vi "To Array U16 1D.vi"(8 "error in":errorcluster, 11 "Generic Image in":refnum<class "Generic Image.lvclass">) -> (0 "error out":errorcluster, 1 "Timestamp":timestamp, 2 "U16":u16[](array[numeric]))   [LabVIEW 2025, in "Generic Image.lvclass"]
uses:
  Generic Image.lvclass
  Generic Image.lvclass/Generic Image.ctl
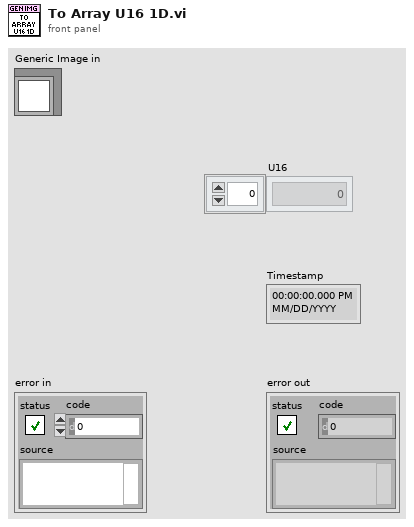
[diagram p1: front panel]
types:
  T1 = typedef "Generic Image.lvclass/Pixel Format.ctl" = enum16{"Grayscale (U8)", "Grayscale (I16)", "Grayscale (SGL)", "Complex (CSG)", "RGB (U32)", "HSL (U32)", "RGB (U64)", "Grayscale (U16)"}
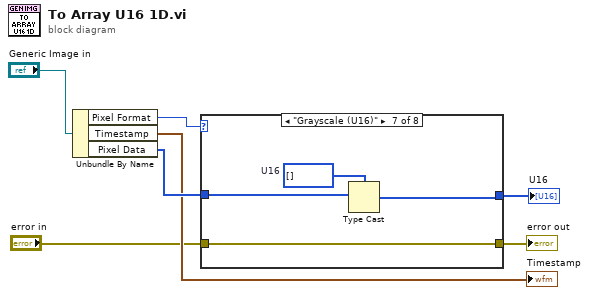
[diagram p0: block diagram]
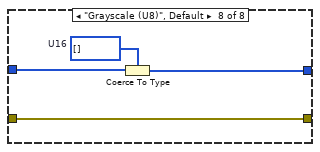
[diagram p8: hidden frame]
diagram:
  n1 = Unbundle By Name("Generic Image in") -> ("Pixel Format"=w5:T1, "Timestamp"=→"Timestamp":timestamp, "Pixel Data"=w6:u8[])
  n2 = case shown="\"Grayscale (U16)\"" w5 {
    tunnel: w6 -> [w8 w10 w12 w14 w16 w18 w23 w27]
    tunnel: "error in" -> [w9 w11 w13 w15 w17 w19 w20 w24]
    tunnel: [w9 w11 w13 w15 w17 w19 w20 w24] -> w2
    tunnel: [w8 w10 w12 w14 w16 w18 w21 w25] -> w1
    frame "Grayscale (I16)" {
    }
    frame "Grayscale (SGL)" {
    }
    frame "Complex (CSG)" {
    }
    frame "RGB (U32)" {
    }
    frame "HSL (U32)" {
    }
    frame "RGB (U64)" {
    }
    frame "Grayscale (U16)" {
      w22 = u16[] []  # U16
      n3 = Type Cast(type=w22, x=w23) -> (*(type *) &x=w21:u16[])
    }
    frame "Grayscale (U8)", Default {
      w26 = u16[] []  # U16
      n4 = Coerce To Type(0:w27, 1:w26) -> (2:w25:u16[])
    }
  }
  "error out" <- w2
  "U16" <- w1
